vi "Untitled 2.vi"() -> ()   [LabVIEW 2020]
uses:
  <vilib>/Analysis/Matrix/Datatypes/RealMatrix.ctl
  <vilib>/Analysis/Matrix/Numeric/Conversions/Matrix To Array - RM.vi
  <vilib>/Analysis/Matrix/NI_Matrix.lvlib
panel:
  out "Real 2D Array":dbl[][](array[numeric])
  out "Predicted State":dbl[][](array[numeric])
  in  "Inputs":T1
  in  "G":T1
  in  "P":T1
  in  "Initial Guess":T1
  in  "H":T1
  in  "R":T1
  in  "Q":T1
  in  "F":T1
  in  "Measurements":T1
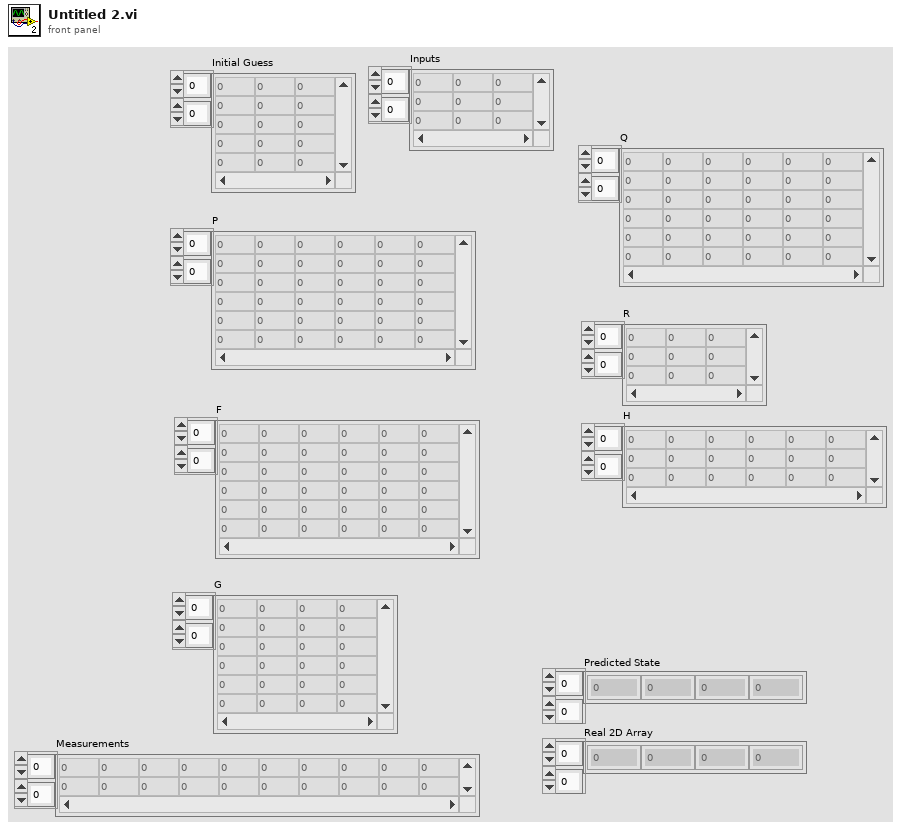
[diagram p1: front panel]
types:
  T1 = typedef "NI_Matrix.lvlib/RealMatrix.ctl" = dbl[][]
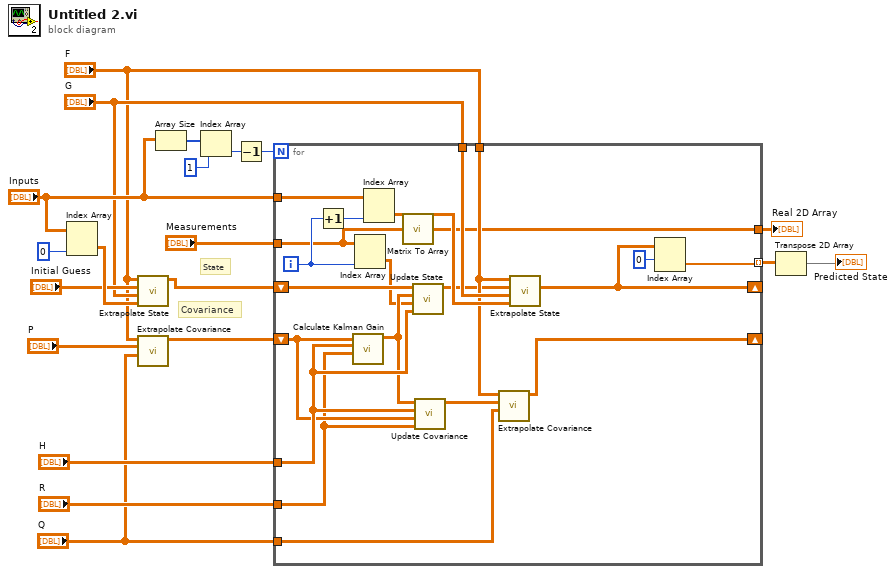
[diagram p0: block diagram]
diagram:
  # "Covariance"
  # "State"
  n1 = Index Array(array="Inputs", index (col)=0) -> (element=w13:T1)  [unwired: 1 in]
  n2 = call "Extrapolate State.vi"("Control"=w13, "G"="G", "Initial State"="Initial Guess", "F"="F") -> ("Predicted State"=w11:T1)  [unwired: 7 in]
  n3 = call "Extrapolate Covariance.vi"("Q"="Q", "Covariance"="P", "F"="F") -> ("New Covariance"=w8:T1)  [unwired: 8 in]
  n4 = Array Size(array="Inputs") -> (size(s)=w17:i32[])
  n5 = Index Array(array=w17, index=1) -> (element=w4:i32)
  n6 = Decrement(x=w4) -> (x-1=w5:i32)
  n7 = for {
    N: w5 -> [_]
    tunnel: "Measurements" -> [w22]
    shift-right: [w25] -> _
    shift-left: w11 -> [w41]
    shift-right: [w31] -> _
    shift-left: w8 -> [w39]
    tunnel: "H" -> [w40]
    tunnel: "R" -> [w38]
    tunnel: "F" -> [w32]
    tunnel: "G" -> [w37]
    tunnel: "Inputs" -> [w36]
    tunnel: "Q" -> [w34]
    tunnel: [w23] -> w3 mode=indexing
    tunnel: [w21] -> w1
    i -> [w26]
    n8 = Increment(x=w26) -> (x+1=w29:i32)
    n9 = call "Calculate Kalman Gain.vi"("R"=w38, "H"=w40, "Prior Covariance"=w39) -> ("Kalman Gain"=w33:T1)  [unwired: 8 in]
    n10 = Index Array(array=w22, index (col)=w26) -> (element=w27:T1)  [unwired: 1 in]
    n11 = Index Array(array=w36, index (col)=w29) -> (element=w35:T1)  [unwired: 1 in]
    n12 = call-poly <vilib>:"Matrix To Array.vi"("Real Matrix"=w22) -> ("Real 2D Array"=w21:dbl[][])
    n13 = call "Update State.vi"("H"=w40, "z"=w27, "K"=w33, "x"=w41) -> ("New State"=w28:T1)  [unwired: 7 in]
    n14 = call "Update Covariance.vi"("R"=w38, "Covariance"=w39, "H"=w40, "K"=w33) -> ("New Covariance"=w30:T1)  [unwired: 7 in]
    n15 = call "Extrapolate Covariance.vi"("Q"=w34, "Covariance"=w30, "F"=w32) -> ("New Covariance"=w31:T1)  [unwired: 8 in]
    n16 = call "Extrapolate State.vi"("Control"=w35, "G"=w37, "Initial State"=w28, "F"=w32) -> ("Predicted State"=w25:T1)  [unwired: 7 in]
    n17 = Index Array(array=w25, index (row)=0) -> (element=w23:dbl[])  [unwired: 1 in]
  }
  "Real 2D Array" <- w1
  n18 = Transpose 2D Array(2D array=w3) -> (transposed array=→"Predicted State":dbl[][])
